vi "removeDuplicateTimes.vi"(8 "error in (no error)":errorcluster, 11 "ScriptEventList in":refnum<class "ScriptEventList.lvclass">) -> (0 "error out":errorcluster, 2 "list":refnum<class "ScriptEventList.lvclass">, 3 "ScriptEventList out":refnum<class "ScriptEventList.lvclass">)   [LabVIEW 2011, in "Tools.lvlib" / "Scripting.lvlib" / "ScriptEventList.lvclass"]
uses:
  ScriptEventList.lvclass
  ScriptEventList.lvclass/ScriptEventList.ctl
  ScriptEvent.lvclass
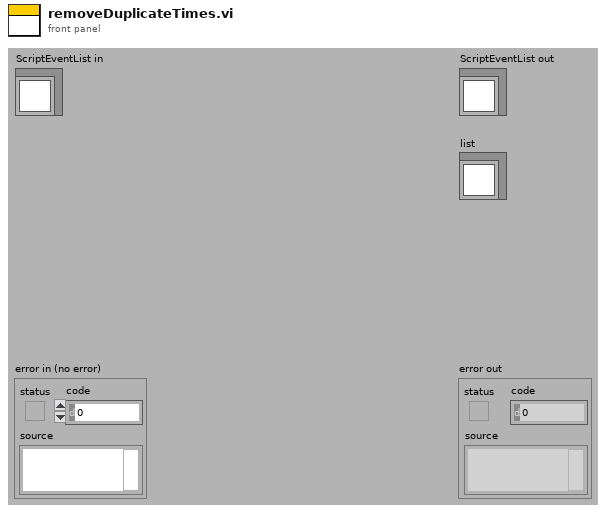
[diagram p1: front panel]
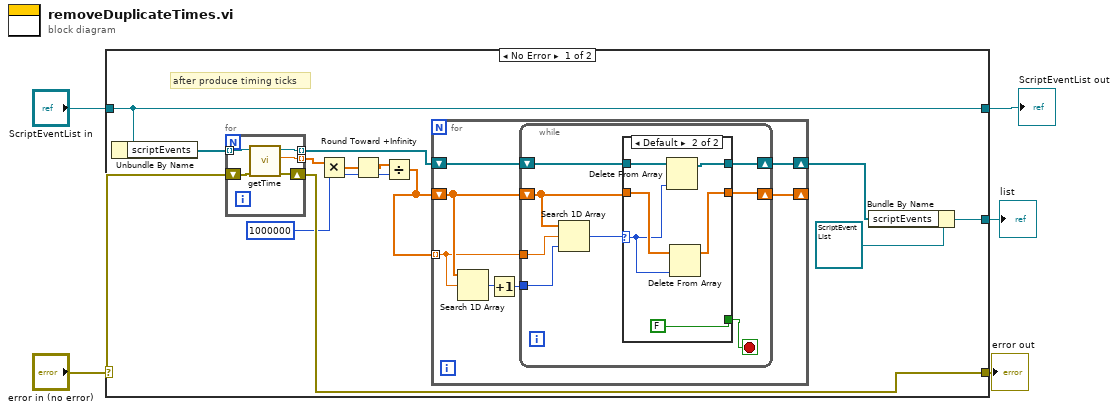
[diagram p0: block diagram]
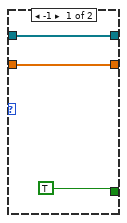
[diagram p2: hidden frame]
diagram:
  n1 = case shown="No Error" "error in (no error)" {
    selector: "error in (no error)" -> [w16 w49]
    tunnel: [w11 w49] -> w4
    tunnel: [w18 w48] -> w2
    tunnel: "ScriptEventList in" -> [w18 w48]
    tunnel: [w12 _] -> w1
    frame No Error {
      w7 = 1000000
      # "after produce timing ticks"
      n2 = Unbundle By Name(w18) -> ("scriptEvents"=w17:refnum<class "ScriptEvent.lvclass">[])
      n3 = for {
        tunnel: w17 -> [w47] mode=indexing
        tunnel: [w45] -> w10 mode=indexing
        tunnel: [w44] -> w15 mode=indexing
        shift-right: [w43] -> w11
        shift-left: w16 -> [w46]
        n4 = call "getTime.vi"("error in (no error)"=w46, "ScriptEvent.lvclass in"=w47) -> ("error out"=w43:errorcluster, "time"=w45:dbl, "ScriptEvent.lvclass out"=w44:refnum<class "ScriptEvent.lvclass">)  [unwired: 7 in]
      }
      n5 = Multiply(x=w10, y=w7) -> (x*y=w9:dbl[])
      n6 = Round Toward +Infinity(x=w9) -> (ceil(x): smallest int >= x=w8:dbl[])
      n7 = Divide(x=w8, y=w7) -> (x/y=w6:dbl[])
      n8 = for {
        tunnel: w6 -> [w23] mode=indexing
        shift-right: [w25] -> _
        shift-left: w6 -> [w24]
        shift-right: [w21] -> w13
        shift-left: w15 -> [w22]
        n9 = Search 1D Array(1D array=w24, element=w23) -> (index of element=w20:i32)  [unwired: 1 in]
        n10 = Increment(x=w20) -> (x+1=w19:i32)
        n11 = while {
          tunnel: w23 -> [w33]
          shift-right: [w27] -> w25
          shift-left: w24 -> [w28]
          tunnel: w19 -> [w26]
          shift-right: [w30] -> w21
          shift-left: w22 -> [w31]
          stop <- w29 stop-if-true
          n12 = Search 1D Array(1D array=w28, element=w33, start index (0)=w26) -> (index of element=w32:i32)
          n13 = case shown="Default" w32 {
            selector: w32 -> [_ w37]
            tunnel: [TRUE FALSE] -> w29
            tunnel: w31 -> [w34 w38]
            tunnel: [w34 w39] -> w30
            tunnel: w28 -> [w35 w41]
            tunnel: [w35 w40] -> w27
            frame -1 {
            }
            frame Default {
              n14 = Delete From Array(array=w38, index=w37) -> (array with subset deleted=w39:refnum<class "ScriptEvent.lvclass">[])  [unwired: 1 in, 1 out]
              n15 = Delete From Array(array=w41, index=w37) -> (array with subset deleted=w40:dbl[])  [unwired: 1 in, 1 out]
            }
          }
        }
      }
      n16 = Bundle By Name(cluster=refnum<class "ScriptEventList.lvclass"> refnum ("ScriptEventList in"), "scriptEvents"=w13) -> (w12:refnum<class "ScriptEventList.lvclass">)
    }
    frame Error {
    }
  }
  "error out" <- w4
  "ScriptEventList out" <- w2
  "list" <- w1
